vi "KepcoDCPwr Abort [TRG].vi"(0 "VISA Session":refnum<visa-resource-name>, 5 "Model In":string, 7 "channel name (\"\")":string="\"\"", 11 "error in (no error)":errorcluster {"code" format="%.0x"}) -> (4 "VISA Session Out":refnum<visa-resource-name>, 6 "Model Out":string, 8 "channel name out (\"\")":string="\"\"" caption="channel name Out (\"\")", 15 "error out":errorcluster {"code" format="%.0x"})   [LabVIEW 2020]
doc: "If the power supply is currently waiting for a trigger to change the output signal, this VI aborts all pending output changes.\n\nIf the power supply is not waiting for a trigger, this VI does nothing and returns VI_SUCCESS."
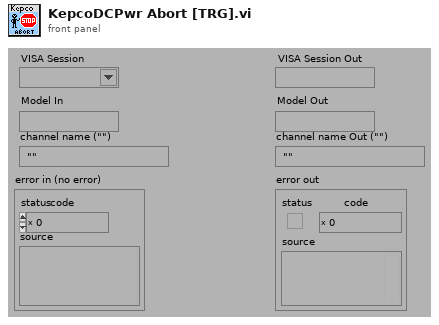
[diagram p1: front panel]
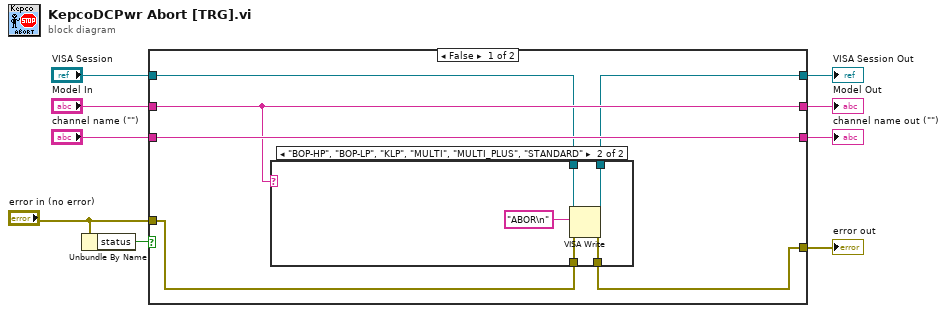
[diagram p0: block diagram]
diagram:
  n1 = Unbundle By Name("error in (no error)") -> ("status"=w8:bool)
  n2 = case shown="False" w8 {
    tunnel: [w11 w26] -> w9
    tunnel: "error in (no error)" -> [w10 w26]
    tunnel: [w12 w25] -> w3
    tunnel: "VISA Session" -> [w13 w25]
    tunnel: [w14 w24] -> w2
    tunnel: "Model In" -> [w14 w24]
    tunnel: [w15 w23] -> w1
    tunnel: "channel name (\"\")" -> [w15 w23]
    frame False {
      n3 = case shown="\"BOP-HP\", \"BOP-LP\", \"KLP\", \"MULTI\", \"MULTI_PLUS\", \"STANDARD\"" w14 {
        tunnel: w10 -> [w16 w21]
        tunnel: w13 -> [w17 w20]
        tunnel: [w17 w19] -> w12
        tunnel: [w16 w18] -> w11
        frame "", Default {
        }
        frame "BOP-HP", "BOP-LP", "KLP", "MULTI", "MULTI_PLUS", "STANDARD" {
          n4 = VISA Write(VISA resource name=w20, write buffer="ABOR\n", error in (no error)=w21) -> (VISA resource name out=w19:refnum<visa-resource-name>, error out=w18:errorcluster)  [unwired: 1 out]
        }
      }
    }
    frame True {
    }
  }
  "error out" <- w9
  "channel name out (\"\")" <- w1
  "Model Out" <- w2
  "VISA Session Out" <- w3
